vi "PH_Waveplate-GUI_6P.PC_SetType.vi"(0 "VI in":refnum<vi>, 2 "Type":T1 items=["Degrees", "Percent"], 5 "error in":errorcluster) -> (14 "VI out":refnum<vi>, 19 "error out":errorcluster)   [LabVIEW 2014, in "PH_Waveplate-GUI_6P.lvlib"]
uses:
  PH_Waveplate-GUI_6P.lvlib
  PH_Waveplate-GUI_6P.Type.ctl
  PH_Basics/PH_Stepmotor_BaseClass/PH_Stepmotor_BaseClass.Axis Information.ctl
  PH_Basics/PH_Stepmotor_BaseClass/PH_Stepmotor_BaseClass.Axis Activity.ctl
  PH_Basics/PH_Stepmotor_BaseClass/PH_Stepmotor_BaseClass.lvlib
  PH_Basics/PH_AxisGUI_BaseClass/PH_AxisGUI_BaseClass.lvlib
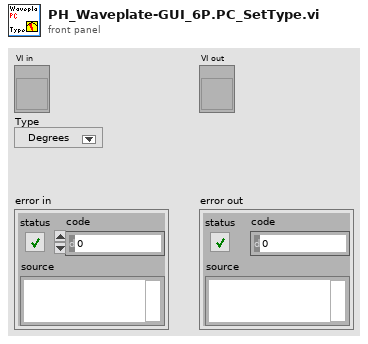
[diagram p1: front panel]
types:
  T1 = typedef "PH_Waveplate-GUI_6P.lvlib/PH_Waveplate-GUI_6P.Type.ctl" = u16
  T2 = typedef "PH_Waveplate-GUI_6P.lvlib/PH_Waveplate-GUI_6P.i attribute.ctl" = cluster{"GUI Refs":cluster{"Meter":refnum<vi>, "Extend Limits":refnum<vi>, "Type":refnum<vi>, "Target":refnum<vi>}, "Extend Waveplate Limit":bool, "Type":T1, "Limit":dbl}
  T3 = typedef "PH_Stepmotor_BaseClass.lvlib/PH_Stepmotor_BaseClass.Axis Information.ctl" = cluster{"Scaled Position":dbl, "Activity":T4}
  T4 = typedef "PH_Stepmotor_BaseClass.lvlib/PH_Stepmotor_BaseClass.Axis Activity.ctl" = enum16{"No Information", "stopped", "running", "Failure", "Alarm", "stopped at backward ES", "stopped at foreward ES"}
  T5 = typedef "PH_AxisGUI_BaseClass.lvlib/PH_AxisGUI_BaseClass.i attribute.ctl" = cluster{"Axes":T6[]}
  T6 = typedef "PH_AxisGUI_BaseClass.lvlib/PH_AxisGUI_BaseClass.Axis Attributes.ctl" = cluster{"Axis GUI Refs":T7, "Address":T8, "Name":string, "Label \"Back\"":string, "Labell \"Forth\"":string, "Moving?":bool}
  T7 = typedef "PH_AxisGUI_BaseClass.lvlib/PH_AxisGUI_BaseClass.Axis GUI Refs.ctl" = cluster{"Back":refnum<vi>, "Forth":refnum<vi>, "Status":refnum<vi>, "Target":refnum<vi>, "Address":refnum<vi>, "Status Bar":refnum<vi>, "Settings":refnum<vi>, "Activity":refnum<vi>, "Clear Error":refnum<vi>}
  T8 = typedef "PH_Stepmotor_BaseClass.lvlib/PH_Stepmotor_BaseClass.Axis Address.ctl" = cluster{"Instance":string, "Motor Nr":i32}
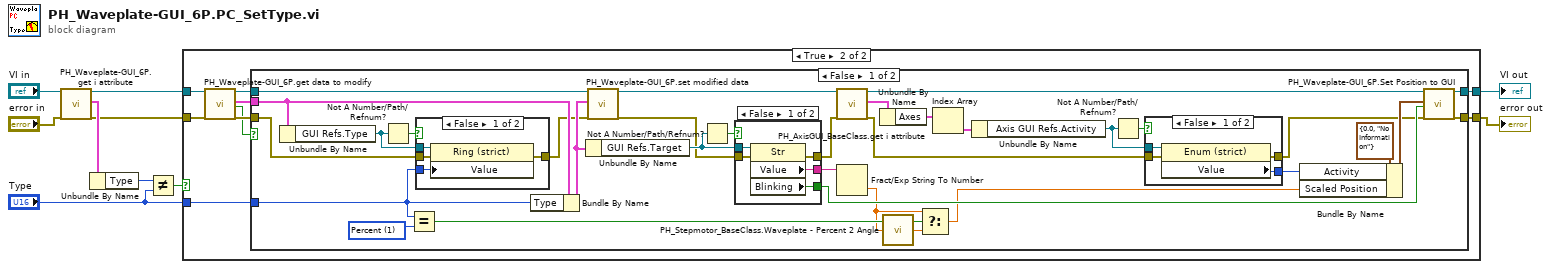
[diagram p0: block diagram]
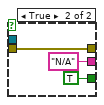
[diagram p3: hidden frame]
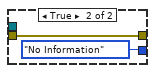
[diagram p4: hidden frame]
diagram:
  n1 = call "PH_Waveplate-GUI_6P.get i attribute.vi"("i ref in"="VI in", "error in (no error)"="error in") -> ("i ref out"=w6:refnum<vi>, "i attribute"=w8:T2, "error out"=w4:errorcluster)  [unwired: 15 in]
  n2 = Unbundle By Name(w8) -> ("Type"=w3:T1)
  n3 = Not Equal?(x=w3, y="Type") -> (x != y?=w1:bool)
  n4 = case shown="True" w1 {
    tunnel: [w12 w14] -> w10
    tunnel: [w11 w13] -> w9
    tunnel: w6 -> [w12 w17]
    tunnel: w4 -> [w11 w16]
    tunnel: "Type" -> [_ w15]
    frame False {
    }
    frame True {
      n5 = call "PH_Waveplate-GUI_6P.get data to modify.vi"("i ref in"=w17, "error in (no error)"=w16) -> ("i ref out"=w21:refnum<vi>, "i attribute"=w19:T2, "timed out"=w18:bool, "error out"=w20:errorcluster)  [unwired: 14 in]
      n6 = case shown="False" w18 {
        tunnel: w15 -> [w27 _]
        tunnel: w19 -> [w53 _]
        tunnel: [w49 w75] -> w14
        tunnel: w21 -> [w54 w75]
        tunnel: [w48 w74] -> w13
        tunnel: w20 -> [w50 w74]
        frame False {
          w26 = T1 1 items=["Degrees", "Percent"] ("y")
          n7 = Unbundle By Name(w53) -> ("GUI Refs.Type"=w51:refnum<vi>)
          n8 = Not A Number/Path/Refnum?(number/path/refnum=w51) -> (NaN/Path/Refnum?=w52:bool)
          n9 = Equal?(x=w27, y=w26) -> (x = y?=w25:bool)
          n10 = case shown="False" w52 {
            tunnel: w50 -> [w72 w73]
            tunnel: [w71 w73] -> w31
            tunnel: w51 -> [w70 _]
            tunnel: w27 -> [w69 _]
            frame False {
              n11 = property class="Ring (strict)"(reference=w70, error in=w72, "Value"=w69) -> (error out=w71:errorcluster)  [unwired: 1 out]
            }
            frame True {
            }
          }
          n12 = Bundle By Name(cluster=w53, "Type"=w27) -> (w47:T2)
          n13 = Unbundle By Name(w47) -> ("GUI Refs.Target"=w32:refnum<vi>)
          n14 = call "PH_Waveplate-GUI_6P.set modified data.vi"("i ref in"=w54, "i attribute"=w47, "error in (no error)"=w31) -> ("i ref out"=w42:refnum<vi>, "error out"=w30:errorcluster)  [unwired: 15 in]
          n15 = Not A Number/Path/Refnum?(number/path/refnum=w32) -> (NaN/Path/Refnum?=w33:bool)
          n16 = case shown="False" w33 {
            tunnel: w30 -> [w59 w62]
            tunnel: [w58 w62] -> w29
            tunnel: w32 -> [w57 _]
            tunnel: [w56 "N/A" ("Value")] -> w44
            tunnel: [w55 TRUE ("Blinking")] -> w43
            frame False {
              n17 = property class="Str"(reference=w57, error in=w59) -> (error out=w58:errorcluster, "Value"=w56:string, "Blinking"=w55:bool)  [unwired: 1 out]
            }
            frame True {
            }
          }
          n18 = call "PH_AxisGUI_BaseClass.get i attribute.vi"("i ref in"=w42, "error in (no error)"=w29) -> ("i ref out"=w41:refnum<vi>, "i attribute"=w40:T5, "error out"=w28:errorcluster)  [unwired: 15 in]
          n19 = Fract/Exp String To Number(string=w44) -> (number=w23:dbl)  [unwired: 3 in, 1 out]
          n20 = Unbundle By Name(w40) -> ("Axes"=w39:T6[])
          n21 = call "PH_Stepmotor_BaseClass.Waveplate - Percent 2 Angle.vi"("rel. Intensity [%]"=w23) -> ("Angle [°]"=w24:dbl)
          n22 = Select(t=w23, s=w25, f=w24) -> (s? t:f=w22:dbl)
          n23 = Index Array(array=w39) -> (element=w38:T6)  [unwired: 1 in]
          n24 = Unbundle By Name(w38) -> ("Axis GUI Refs.Activity"=w34:refnum<vi>)
          n25 = Not A Number/Path/Refnum?(number/path/refnum=w34) -> (NaN/Path/Refnum?=w35:bool)
          n26 = case shown="False" w35 {
            tunnel: w34 -> [w66 _]
            tunnel: [w65 w68] -> w37
            tunnel: [w64 PH_Stepmotor_BaseClass.Axis_Activity."No Information" ("Value")] -> w36
            tunnel: w28 -> [w63 w68]
            frame False {
              n27 = property class="Enum (strict)"(reference=w66, error in=w63) -> (error out=w65:errorcluster, "Value"=w64:T4)  [unwired: 1 out]
            }
            frame True {
            }
          }
          n28 = Bundle By Name(cluster=T3 {"Scaled Position"=0.0, "Activity"=enum."No Information"} ("Information"), "Activity"=w36, "Scaled Position"=w22) -> (w45:T3)
          n29 = call "PH_Waveplate-GUI_6P.Set Position to GUI.vi"("i ref in"=w41, "Axis Information"=w45, "no link"=w43, "error in"=w37) -> ("i ref out"=w49:refnum<vi>, "error out"=w48:errorcluster)  [unwired: 14 in]
        }
        frame True {
        }
      }
    }
  }
  "VI out" <- w10
  "error out" <- w9
